vi "Add-filtered-data-to-report.vi"(8 "error in":errorcluster, 9 "Filter params. ref. in":refnum<data-value>, 10 "Storage element in":T1 {"Temperature characteristics"."Stand. dev. temperature" format="%#.1f"; "Temperature characteristics"."Min. temperature" format="%#.0f"; "Temperature characteristics"."Max. temperature" format="%#.0f"; "Temperature characteristics"."Average temperature" format="%#.0f"}, 11 "Storage params. ref. in":refnum<data-value>) -> (0 "error IO":errorcluster, 1 "Filter params. ref.":refnum<data-value>, 2 "Storage element":T1 {"Temperature characteristics"."Stand. dev. temperature" format="%#.1f"; "Temperature characteristics"."Min. temperature" format="%#.0f"; "Temperature characteristics"."Max. temperature" format="%#.0f"; "Temperature characteristics"."Average temperature" format="%#.0f"}, 3 "Storage params. ref.":refnum<data-value>)   [LabVIEW 2013, in "CameraVision.lvlib" / "CV-Filter.lvclass"]
uses:
  CV-Filter.lvclass
  Storage/CV-Storage.lvclass
  Buffers/Storage-buffer.ctl
  <vilib>/vision/Image Controls.llb/IMAQ Image.ctl
  Temperature/Temperature-characteristics.ctl
  Analysis/Characteristics-cluster.ctl
  Storage/CV-Storage.lvclass/CV-Storage.ctl
  CV-Filter.lvclass/CV-Filter.ctl
  UI/Module-states.ctl
  Write Filter status.vi
  Storage/Read Camera suffix.vi
  Read Filter file reference.vi
  Read Filter file labels.vi
  Read Values temp.vi
  UI/CV-UI.lvclass
  Temperature/CV-Temperature.lvclass
  Analysis/CV-Analysis.lvclass
  Buffers/CV-Buffers.lvclass
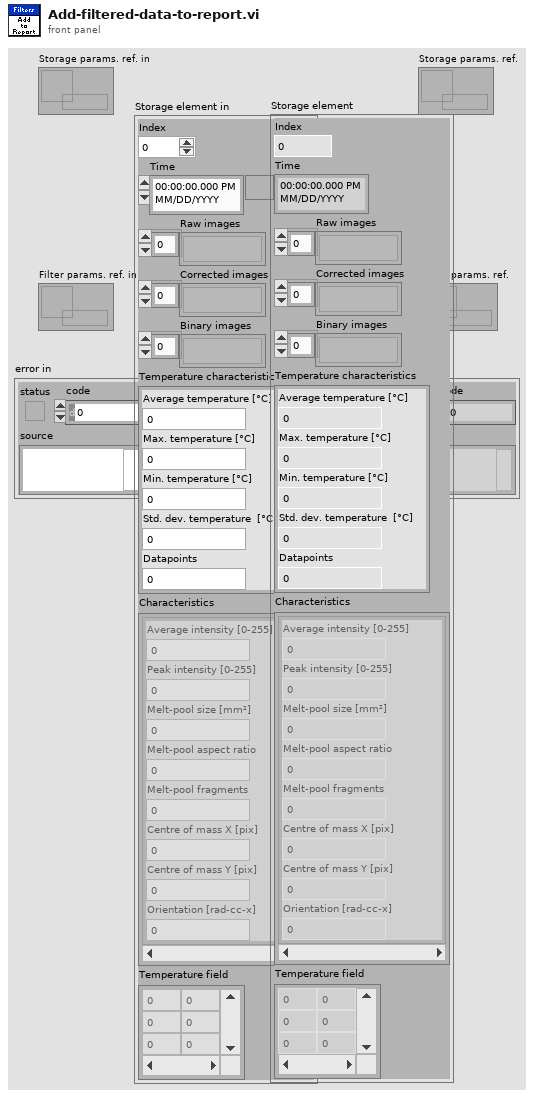
[diagram p1: front panel]
types:
  T1 = typedef "CameraVision.lvlib/CV-Buffers.lvclass/Storage-buffer.ctl" = cluster{"Index":i32, "Time":timestamp, "Raw images":T2[], "Corrected images":T2[], "Binary images":T2[], "Temperature characteristics":T3, "Characteristics":T4[], "Temperature field":dbl[][]}
  T2 = typedef "IMAQ Image.ctl" = refnum<image>
  T3 = typedef "CameraVision.lvlib/CV-Temperature.lvclass/Temperature-characteristics.ctl" = cluster{"Average temperature ":dbl, "Max. temperature":dbl, "Min. temperature":dbl, "Stand. dev. temperature":dbl, "Datapoints":dbl}
  T4 = typedef "CameraVision.lvlib/CV-Analysis.lvclass/Characteristics-cluster.ctl" = cluster{"Average intensity":dbl, "Peak intensity":dbl, "Melt-pool size":dbl, "Melt-pool aspect ratio":dbl, "Melt-pool fragments":dbl, "Centre of mass X":dbl, "Centre of mass Y":dbl, "Orientation":dbl}
  T5 = typedef "CameraVision.lvlib/CV-UI.lvclass/Module-states.ctl" = enum16{"Inactive", "Active", "Data-loss", "Error", "Simulation", "Synchronizing", "Initialized", "Released"}
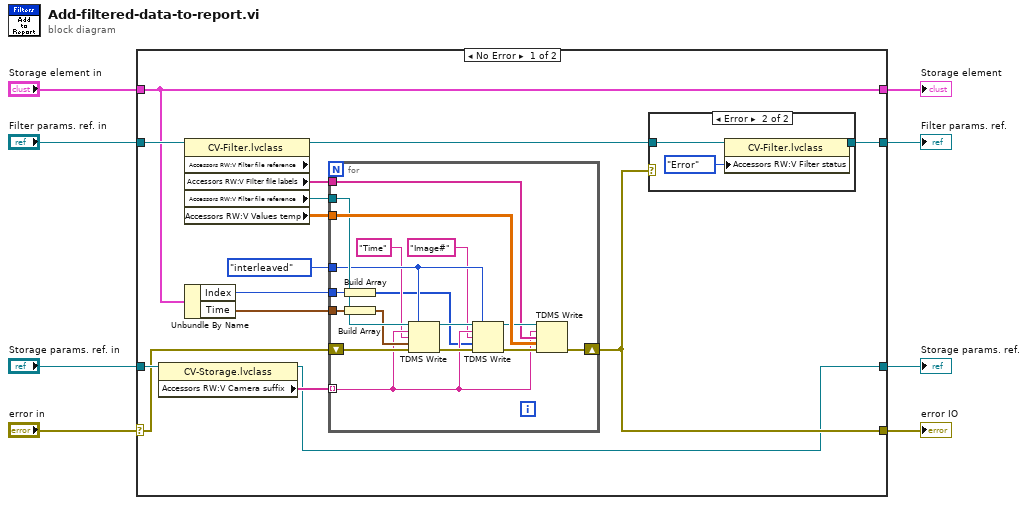
[diagram p0: block diagram]
diagram:
  n1 = case shown="No Error" "error in" {
    selector: "error in" -> [w15 w47]
    tunnel: "Filter params. ref. in" -> [w23 w48]
    tunnel: [w20 w48] -> w6
    tunnel: [w14 w47] -> w5
    tunnel: "Storage element in" -> [w10 w46]
    tunnel: "Storage params. ref. in" -> [w22 w45]
    tunnel: [w10 w46] -> w2
    tunnel: [w9 w45] -> w1
    frame No Error {
      n2 = property class="CV-Storage.lvclass"(reference=w22) -> (reference out=w9:refnum<data-value>, "Accessors RW:V Camera suffix"=w21:string[])  [unwired: 1 in, 1 out]
      n3 = property class="CV-Filter.lvclass" props=["Accessors RW:V Filter file reference", "Accessors RW:V Filter file labels", "Accessors RW:V Filter file reference", "Accessors RW:V Values temp"](reference=w23) -> (reference out=w13:refnum<data-value>, "Accessors RW:V Filter file labels"=w19:string[], "Accessors RW:V Filter file reference"=w11:refnum<k34>, "Accessors RW:V Values temp"=w12:dbl[][])  [unwired: 1 in, 2 out]
      n4 = Unbundle By Name(w10) -> ("Index"=w16:i32, "Time"=w17:timestamp)
      n5 = for {
        tunnel: w21 -> [w28] mode=indexing
        tunnel: w19 -> [w29]
        tunnel: w11 -> [w37]
        shift-right: [w40] -> w14
        shift-left: w15 -> [w38]
        tunnel: w12 -> [w39]
        tunnel: w17 -> [w36]
        tunnel: enum16{"decimated", "interleaved"}."interleaved" ("data layout (0:decimated)") -> [w33]
        tunnel: w16 -> [w24]
        n6 = Build Array(w24) -> (w25:i32[])
        n7 = Build Array(w36) -> (w35:timestamp[])
        n8 = TDMS Write(0:w37, 1:w33, 5:w28, 7:"Time", 9:w35, 11:w38) -> (4:w34:refnum<k34>, 15:w32:errorcluster)  [unwired: 2 out]
        n9 = TDMS Write(0:w34, 1:w33, 5:w28, 7:"Image#", 9:w25, 11:w32) -> (4:w30:refnum<k34>, 15:w31:errorcluster)  [unwired: 2 out]
        n10 = TDMS Write(0:w30, 5:w28, 7:w29, 9:w39, 11:w31) -> (15:w40:errorcluster)  [unwired: 1 in, 3 out]
      }
      n11 = case shown="Error" w14 {
        tunnel: w13 -> [w41 w44]
        tunnel: [w41 w43] -> w20
        frame No Error {
        }
        frame Error {
          n12 = property class="CV-Filter.lvclass"(reference=w44, "Accessors RW:V Filter status"=Module-states."Error" ("Filter status")) -> (reference out=w43:refnum<data-value>)  [unwired: 1 in, 1 out]
        }
      }
    }
    frame Error {
    }
  }
  "Filter params. ref." <- w6
  "error IO" <- w5
  "Storage params. ref." <- w1
  "Storage element" <- w2
